vi "Format_To_Chart.vi"(8 "error in (no error)":errorcluster, 10 "Temperature Data in":sgl[][](array[numeric])) -> (0 "error out":errorcluster, 1 "Motor Temperature Data":waveform(dbl)[](array[waveform]), 2 "Bearing Temperature Data":waveform(dbl)[](array[waveform]), 3 "Bearing Temp Data":T2, 5 "Channel (24 - 31)":T3, 7 "Motor Temp Data":T1)   [LabVIEW 2019, in "MHL.lvlib"]
uses:
  MHL.lvlib
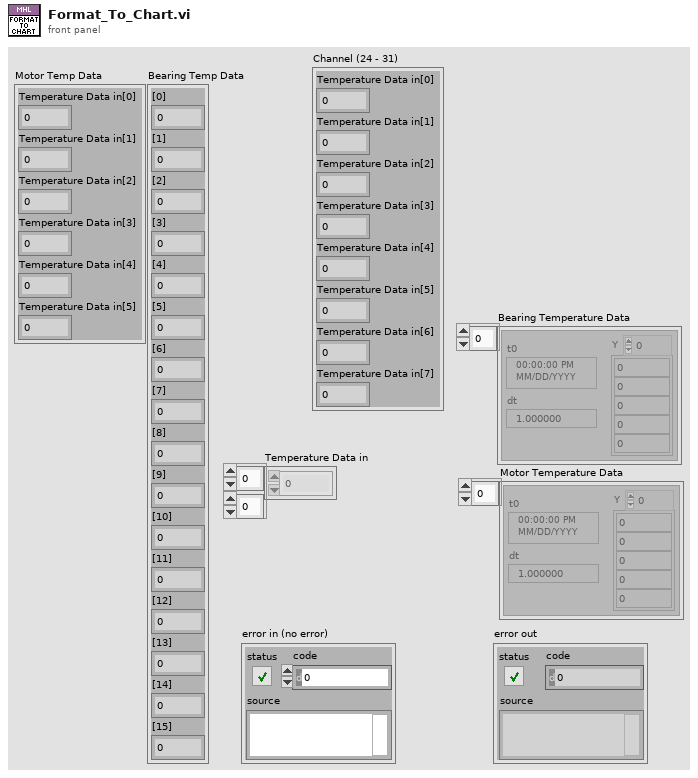
[diagram p1: front panel]
types:
  T1 = cluster{"Temperature Data in[0]":sgl, "Temperature Data in[1]":sgl, "Temperature Data in[2]":sgl, "Temperature Data in[3]":sgl, "Temperature Data in[4]":sgl, "Temperature Data in[5]":sgl}
  T2 = cluster{"[0]":sgl, "[1]":sgl, "[2]":sgl, "[3]":sgl, "[4]":sgl, "[5]":sgl, "[6]":sgl, "[7]":sgl, "[8]":sgl, "[9]":sgl, "[10]":sgl, "[11]":sgl, "[12]":sgl, "[13]":sgl, "[14]":sgl, "[15]":sgl}
  T3 = cluster{"Temperature Data in[0]":sgl, "Temperature Data in[1]":sgl, "Temperature Data in[2]":sgl, "Temperature Data in[3]":sgl, "Temperature Data in[4]":sgl, "Temperature Data in[5]":sgl, "Temperature Data in[6]":sgl, "Temperature Data in[7]":sgl}
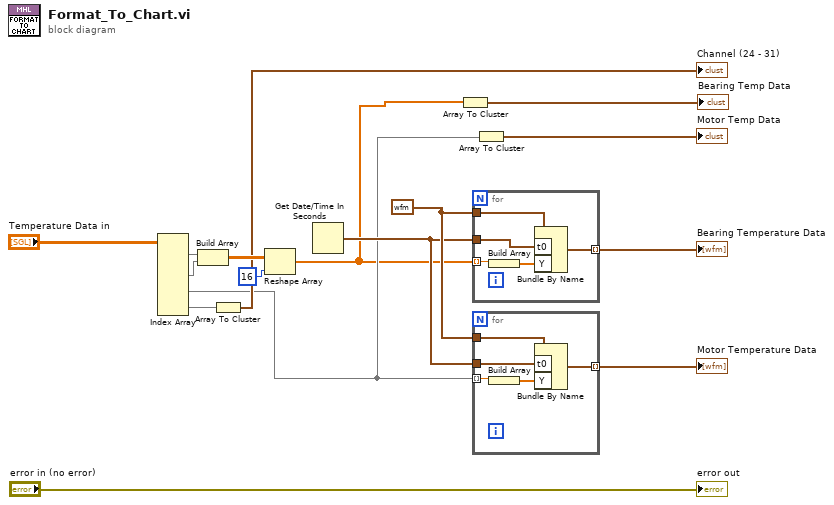
[diagram p0: block diagram]
diagram:
  w9 = waveform(dbl) {"t0"=timestamp(0 s since 1904-01-01), "dt"=1.0, "Y"=[]} ("waveform")
  n1 = Index Array(array="Temperature Data in") -> (element #1=w14:sgl[], element #2=w15:sgl[], element #3=w2:sgl[], element #4=w6:sgl[])  [unwired: 8 in]
  n2 = Build Array(w14, w15) -> (w16:sgl[][])
  n3 = Array To Cluster(array=w6) -> (cluster=→"Channel (24 - 31)":T3)
  n4 = Reshape Array(w16, 16 ("dimension size")) -> (w1:sgl[])
  n5 = Get Date/Time In Seconds() -> (seconds since 1Jan1904=w7:timestamp)
  n6 = Array To Cluster(array=w1) -> (cluster=→"Bearing Temp Data":T2)
  n7 = for {
    tunnel: w7 -> [w21]
    tunnel: w9 -> [w20]
    tunnel: [w19] -> w11 mode=indexing
    tunnel: w1 -> [w18] mode=indexing
    n8 = Build Array(w18) -> (w17:sgl[])
    n9 = Bundle By Name(cluster=w20, "t0"=w21, "Y"=w17) -> (w19:waveform(dbl))
  }
  "Bearing Temperature Data" <- w11
  n10 = for {
    tunnel: w7 -> [w26]
    tunnel: w9 -> [w25]
    tunnel: [w24] -> w8 mode=indexing
    tunnel: w2 -> [w23] mode=indexing
    n11 = Build Array(w23) -> (w22:sgl[])
    n12 = Bundle By Name(cluster=w25, "t0"=w26, "Y"=w22) -> (w24:waveform(dbl))
  }
  "Motor Temperature Data" <- w8
  n13 = Array To Cluster(array=w2) -> (cluster=→"Motor Temp Data":T1)
  "error out" <- "error in (no error)"
